vi "programa 1.vi"() -> ()   [LabVIEW 2011]
panel:
  out "multiplicacion":dbl
  out "division":dbl
  out "resta":dbl
  out "suma":dbl
  in  "numero2":dbl
  in  "numero1":dbl
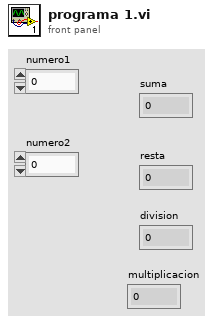
[diagram p1: front panel]
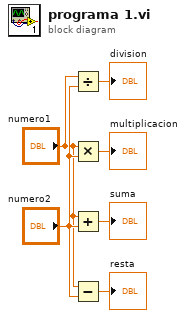
[diagram p0: block diagram]
diagram:
  n1 = Divide(x="numero1", y="numero2") -> (x/y=→"division":dbl)
  n2 = Multiply(x="numero1", y="numero2") -> (x*y=→"multiplicacion":dbl)
  n3 = Add(x="numero1", y="numero2") -> (x+y=→"suma":dbl)
  n4 = Subtract(x="numero1", y="numero2") -> (x-y=→"resta":dbl)
